vi "Sr530 Autoscale.vi"(4 "error in":errorcluster, 7 "Ressource VISA":refnum<visa-resource-name>="GPIB0::8::INSTR") -> (0 "error out":errorcluster, 1 "Sensitivity":u16(ring)=1 items=["10 nV"=1, "20 nV"=2, "50 nV"=3, "100 nV"=4, "200 nV"=5, "500 nV"=6, "1 µV"=7, "2 µV"=8, "5 µV"=9, "10 µV"=10, "20 µV"=11, "50 µV"=12, "100µV"=13, "200 µV"=14, "500µV"=15, "1 mV"=16, "2 mV"=17, "5 mV"=18, "10 mV"=19, "20 mV"=20, "50 mV"=21, "100 mV"=22], 2 "OverRanged":bool, 3 "Ressource VISA Out":refnum<visa-resource-name>="GPIB0::8::INSTR")   [LabVIEW 2019]
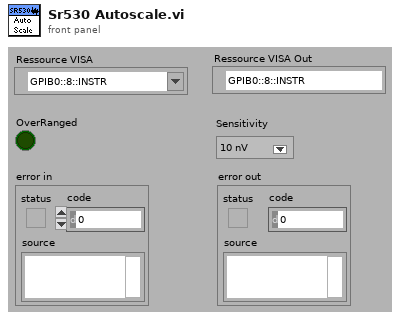
[diagram p1: front panel]
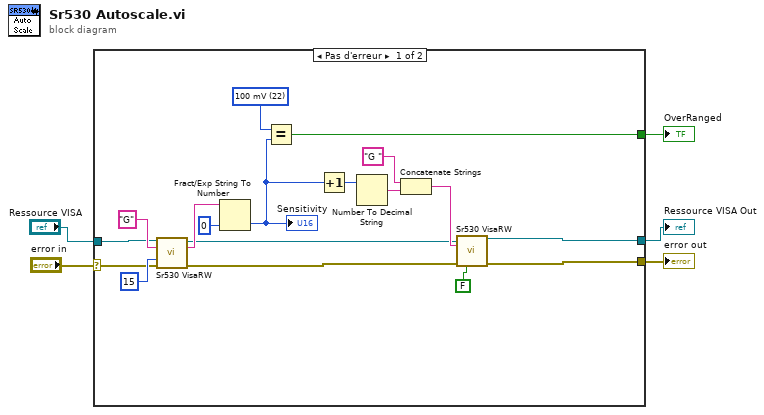
[diagram p0: block diagram]
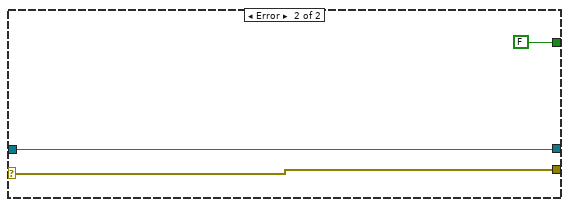
[diagram p2: hidden frame]
diagram:
  n1 = case shown="Pas d'erreur" "error in" {
    selector: "error in" -> [w18 w26]
    tunnel: [w9 w26] -> w5
    tunnel: [w11 FALSE] -> w4
    tunnel: "Ressource VISA" -> [w19 w24]
    tunnel: [w10 w24] -> w1
    frame No Error {
      w8 = u16 22 items=["10 nV"=1, "20 nV"=2, "50 nV"=3, "100 nV"=4, "200 nV"=5, "500 nV"=6, "1 µV"=7, "2 µV"=8, "5 µV"=9, "10 µV"=10, "20 µV"=11, "50 µV"=12, "100µV"=13, "200 µV"=14, "500µV"=15, "1 mV"=16, "2 mV"=17, "5 mV"=18, "10 mV"=19, "20 mV"=20, "50 mV"=21, "100 mV"=22] ("Sensitivity")
      n2 = call <userlib>:"Sr530 VisaRW.vi"("VISA Rsrc"=w19, "ChaineCom"="G", "Nbcaract"=u32 15, "error in (no error)"=w18) -> ("VISA Rsrc Out"=w12:refnum<visa-resource-name>, "ChaineRep"=w21:string, "error out"=w13:errorcluster)  [unwired: 6 in, 3 out]
      n3 = Fract/Exp String To Number(string=w21, default (0 dbl)=u16 0 ("valeur par défaut (0 I32)")) -> (number=w6:u16)  [unwired: 2 in, 1 out]
      "Sensitivity" <- w6
      n4 = Equal?(x=w8, y=w6) -> (x = y?=w11:bool)
      n5 = Increment(x=w6) -> (x+1=w7:u16)
      n6 = Number To Decimal String(number=w7) -> (decimal integer string=w16:string)  [unwired: 1 in]
      n7 = Concatenate Strings("G " ("ChaineCom"), w16) -> (w14:string)
      n8 = call <userlib>:"Sr530 VisaRW.vi"("VISA Rsrc"=w12, "ChaineCom"=w14, "error in (no error)"=w13, "Lecture?(T)"=FALSE) -> ("VISA Rsrc Out"=w10:refnum<visa-resource-name>, "error out"=w9:errorcluster)  [unwired: 6 in, 4 out]
    }
    frame Error {
    }
  }
  "error out" <- w5
  "OverRanged" <- w4
  "Ressource VISA Out" <- w1
